vi "onCreate.vi"(8 "error in (no error)":errorcluster, 11 "Server in":refnum<class "Server.lvclass">) -> (0 "error out":errorcluster, 3 "Server out":refnum<class "Server.lvclass">)   [LabVIEW 2013, in "MQTT Server.lvlib" / "Server.lvclass"]
uses:
  Server.lvclass
  SessionRef -- cluster.ctl
  MQTT_Base/Base Class/Response -- cluster.ctl
  <vilib>/LabVIEW Open Source Project/MQTT Control Packets/Control Packets/ControlPacket/ControlPacket.lvclass
  MQTT_Base/Base Class/MQTT_Base.lvclass
  Server.lvclass/Server.ctl
  StoredSessions/StoredSessions.lvclass
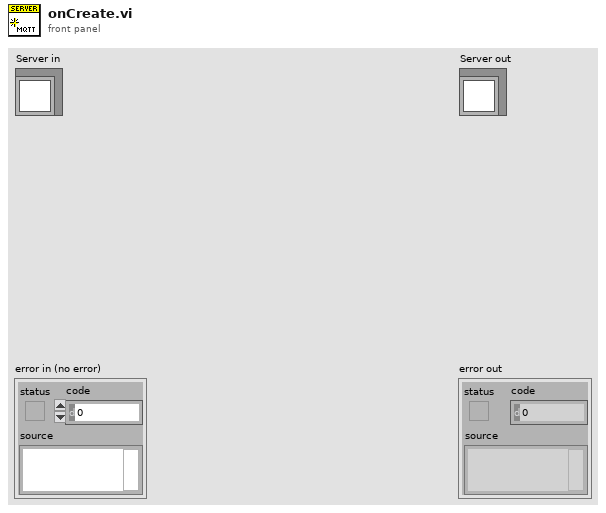
[diagram p1: front panel]
types:
  T1 = typedef "MQTT Server.lvlib/Server.lvclass/SessionRef -- cluster.ctl" = cluster{"ClientID":string, "SessionMailbox":refnum<queue>}
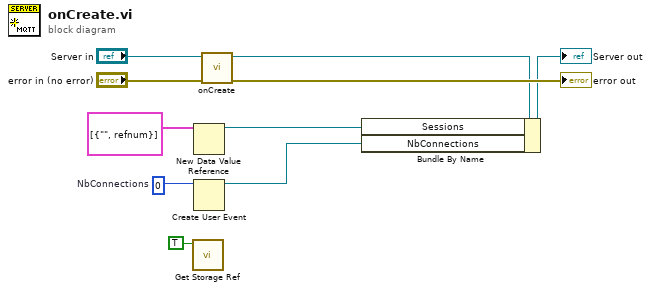
[diagram p0: block diagram]
diagram:
  w4 = u32 0  # NbConnections
  n1 = call "Get Storage Ref.vi"("Init (F)"=TRUE) -> ()  [unwired: 10 in, 1 out]
  n2 = New Data Value Reference(data value=T1[] [{"ClientID"="", "SessionMailbox"=refnum}]) -> (data value reference=w6:refnum<data-value>)  [unwired: 1 in, 1 out]
  n3 = Create User Event(user event datatype=w4) -> (user event=w3:refnum<user-event>)  [unwired: 1 in, 1 out]
  n4 = call-parent "onCreate.vi"("error in (no error)"="error in (no error)", "MQTT_Base in"="Server in") -> ("error out"=→"error out":errorcluster, "MQTT_Base out"=w5:refnum<class "Server.lvclass">)  [unwired: 8 in]
  n5 = Bundle By Name(cluster=w5, "Sessions"=w6, "NbConnections"=w3) -> (→"Server out":refnum<class "Server.lvclass">)
